vi "Add Analyser.vi"(0 "Microscope in":refnum<class "Microscope.lvclass">, 5 "Label":string, 7 "Analyser":refnum<class "Analyser.lvclass">, 9 "RegisterInPipleline?(F)":bool=TRUE, 11 "error in (no error)":errorcluster) -> (4 "Microscope out":refnum<class "Microscope.lvclass">, 6 "key already included?":bool, 8 "value unchanged?":bool, 15 "error out":errorcluster)   [LabVIEW 2020, in "Microscope.lvlib" / "Microscope.lvclass"]
uses:
  Microscope.lvclass
  C:/Program Files/National Instruments/LabVIEW 2020/vi.lib/ActorFramework/Actor/Actor.lvclass
  Analyser/Analyser/Analyser.lvclass
  Microscope.lvclass/Microscope.ctl
  <vilib>/ActorFramework/Actor/Actor.lvclass
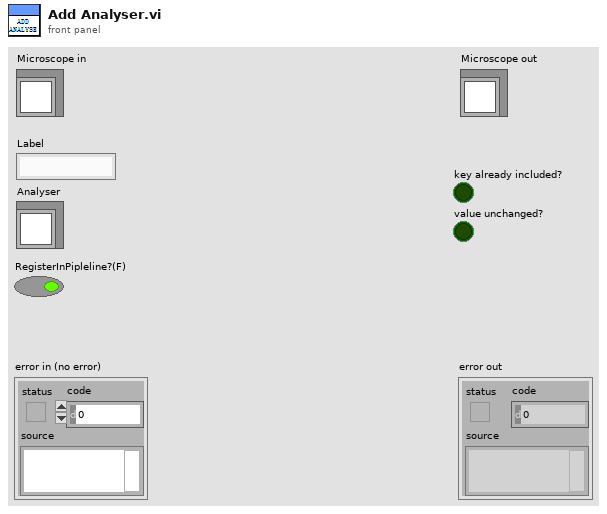
[diagram p1: front panel]
types:
  T1 = map{string, refnum<class "Message Enqueuer.lvclass">}
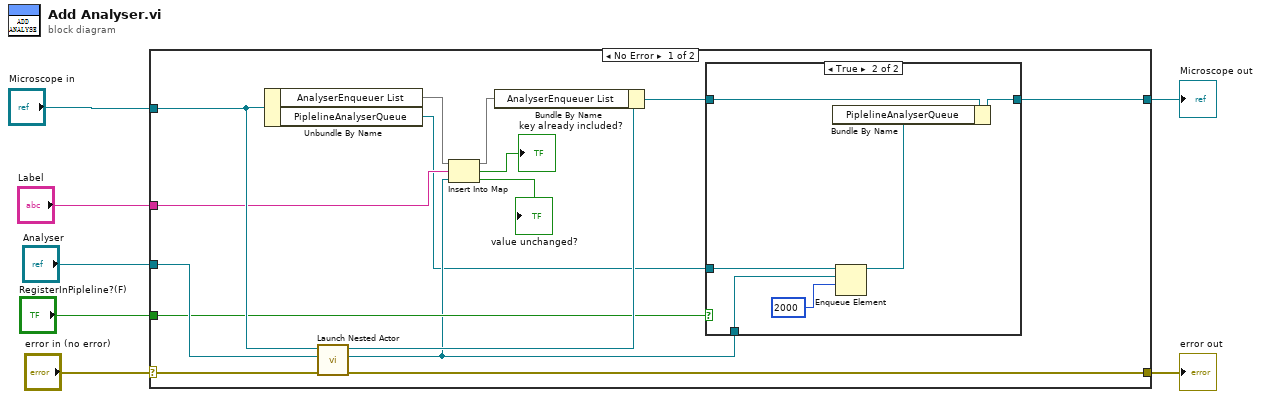
[diagram p0: block diagram]
diagram:
  n1 = case shown="No Error" "error in (no error)" {
    selector: "error in (no error)" -> [w22 w31]
    tunnel: [w21 w31] -> w6
    tunnel: [w8 w30] -> w4
    tunnel: "Microscope in" -> [w18 w30]
    tunnel: "Analyser" -> [w19 _]
    tunnel: "Label" -> [w16 _]
    tunnel: "RegisterInPipleline?(F)" -> [w12 _]
    frame No Error {
      n2 = Unbundle By Name(w18) -> ("AnalyserEnqueuer List"=w17:T1, "PiplelineAnalyserQueue"=w9:refnum<queue>)
      n3 = call <vilib>:"Launch Nested Actor.vi"("error in (no error)"=w22, "Nested Actor"=w19, "Caller Actor in"=w18) -> ("error out"=w21:errorcluster, "Nested Actor's Enqueuer"=w10:refnum<class "Message Enqueuer.lvclass">, "Caller Actor out"=w20:refnum<class "Microscope.lvclass">)  [unwired: 6 in]
      n4 = Insert Into Map(map in=w17, key=w16, value=w10) -> (map out=w15:T1, key already included?=→"key already included?":bool, value unchanged?=→"value unchanged?":bool)
      n5 = Bundle By Name(cluster=w20, "AnalyserEnqueuer List"=w15) -> (w11:refnum<class "Microscope.lvclass">)
      n6 = case shown="True" w12 {
        tunnel: w11 -> [w23 w26]
        tunnel: w10 -> [_ w28]
        tunnel: w9 -> [_ w29]
        tunnel: [w23 w25] -> w8
        frame False {
        }
        frame True {
          n7 = Enqueue Element(queue=w29, element=w28, timeout in ms (-1)=2000) -> (queue out=w24:refnum<queue>)  [unwired: 1 in, 2 out]
          n8 = Bundle By Name(cluster=w26, "PiplelineAnalyserQueue"=w24) -> (w25:refnum<class "Microscope.lvclass">)
        }
      }
    }
    frame Error {
    }
  }
  "error out" <- w6
  "Microscope out" <- w4
